vi "240920.vi"() -> ()   [LabVIEW 2024]
panel:
  out "Array 3":bool[](array[boolean])
  out "Array 2":bool[](array[boolean])
  in  "Numeric 2":dbl
  in  "Numeric":dbl
  out "Boolean 3":bool
  in  "Boolean 2":bool
  out "Array":bool[](array[boolean])
  in  "Boolean":bool
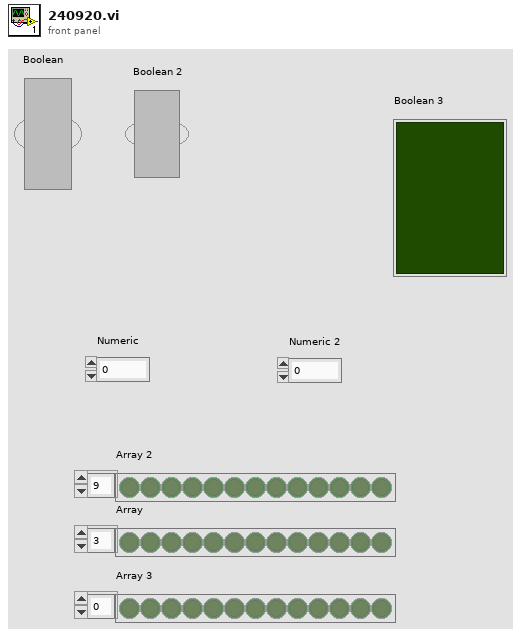
[diagram p1: front panel]
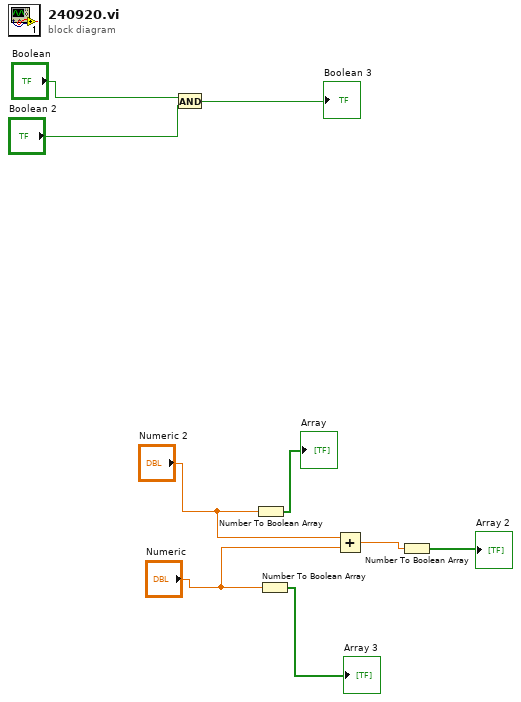
[diagram p0: block diagram]
diagram:
  n1 = And(x="Boolean", y="Boolean 2") -> (x .and. y?=→"Boolean 3":bool)
  n2 = Number To Boolean Array(number="Numeric 2") -> (Boolean array=→"Array":bool[])
  n3 = Number To Boolean Array(number="Numeric") -> (Boolean array=→"Array 3":bool[])
  n4 = Add(x="Numeric 2", y="Numeric") -> (x+y=w3:dbl)
  n5 = Number To Boolean Array(number=w3) -> (Boolean array=→"Array 2":bool[])
